vi "run.update_set_property.vi"(8 "error in":errorcluster, 11 "RunUpdateStaging in":refnum<class "RunUpdateStaging.lvclass">) -> (0 "error out":errorcluster, 3 "RunUpdateStaging out":refnum<class "RunUpdateStaging.lvclass">)   [LabVIEW 2020, in "RunUpdateStaging.lvclass"]
doc: "Sets a property on the staged update, replacing the run's entire property set with the accumulated properties when applied."
uses:
  RunUpdateStaging.lvclass
  RunUpdateStaging.lvclass/RunUpdateStaging.ctl
  client.lvlib
panel:
  in  "key":string
  in  "value":string
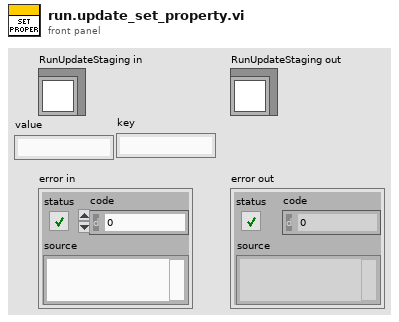
[diagram p1: front panel]
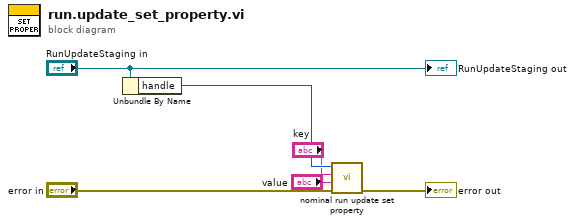
[diagram p0: block diagram]
diagram:
  n1 = Unbundle By Name("RunUpdateStaging in") -> ("handle"=w4:i32)
  n2 = call "nominal run update set property.vi"("error in (no error)"="error in", "value"="value", "key"="key", "staging"=w4) -> ("error out"=→"error out":errorcluster)  [unwired: 6 in, 1 out]
  "RunUpdateStaging out" <- "RunUpdateStaging in"
